vi "GE 5565PIORC.Registers.LISR.Auto Clear Flag.Get.vi"(8 "error in (no error)":errorcluster, 11 "GE 5565PIORC in":refnum<class "GE 5565PIORC.lvclass">) -> (0 "error out":errorcluster, 2 "Auto Clear Flag":bool, 3 "GE 5565PIORC out":refnum<class "GE 5565PIORC.lvclass">)   [LabVIEW 2020, in "GE 5565PIORC.lvclass"]
doc: "This bit is a read-only status indicator of the corresponding bit in the LIER Register. When this bit is high (1), the Global Interrupt Enable (Bit 14) will automatically be cleared as this register (LISR) is being read. Clearing the Global Interrupt Enable de-asserts the LINTi# and, in turn, releases the PCI Interrupt."
uses:
  GE 5565PIORC.lvclass
  GE 5565PIORC.Registers.RFM Control and Status.ctl
  GE 5565PIORC.lvclass/GE 5565PIORC.ctl
  GE 5565PIORC.Registers.RFM Control and Status.Read (U32).vi
  Methods/GE 5565PIORC.Bit Manipulation.Get Bit (U32).vi
  Methods/GE 5565PIORC.Registers.Read.vi
  Methods/GE 5565PIORC.Registers.Read (U32).vi
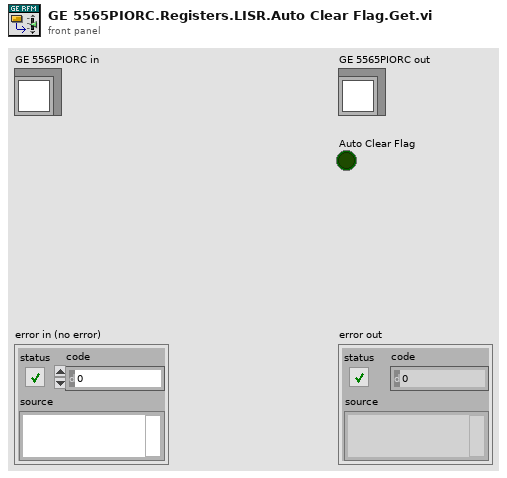
[diagram p1: front panel]
types:
  T1 = typedef "GE 5565PIORC.lvclass/GE 5565PIORC.Registers.RFM Control and Status.ctl" = u32
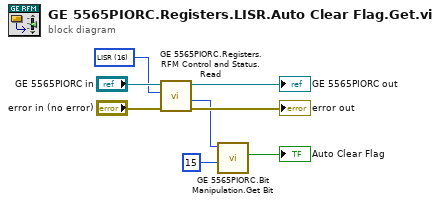
[diagram p0: block diagram]
diagram:
  w4 = T1 16 items=["BRV"=0, "BID"=1, "BRB"=2, "NID"=4, "LCSR1"=8, "LISR"=16, "LIER"=20, "NTD"=24, "NTN"=28, "NIC"=29, "ISD1"=32, "SID1"=36, "ISD2"=40, "SID2"=44, "ISD3"=48, "SID3"=52, "ISD4"=56, "SID4"=60] ("Register")
  n1 = call-poly "GE 5565PIORC.Registers.RFM Control and Status.Read.vi"("error in (no error)"="error in (no error)", "Register"=w4, "GE 5565PIORC in"="GE 5565PIORC in") -> ("error out"=→"error out":errorcluster, "Value"=w3:u32, "GE 5565PIORC out"=→"GE 5565PIORC out":refnum<class "GE 5565PIORC.lvclass">)  [unwired: 6 in]
  n2 = call-poly "GE 5565PIORC.Bit Manipulation.Get Bit.vi"("bit index"=15, "packed value in"=w3) -> ("bit"=→"Auto Clear Flag":bool)  [unwired: 8 in, 1 out]
